vi "PulseProtocol.vi"(11 "Array":string[](array[string])) -> (0 "y2Pulse":i32, 1 "y1Pulse":i32, 2 "xPulse":i32, 3 "modePulse":string)   [LabVIEW 2018]
uses:
  Global Variables.vi
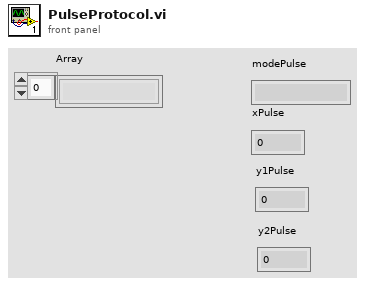
[diagram p1: front panel]
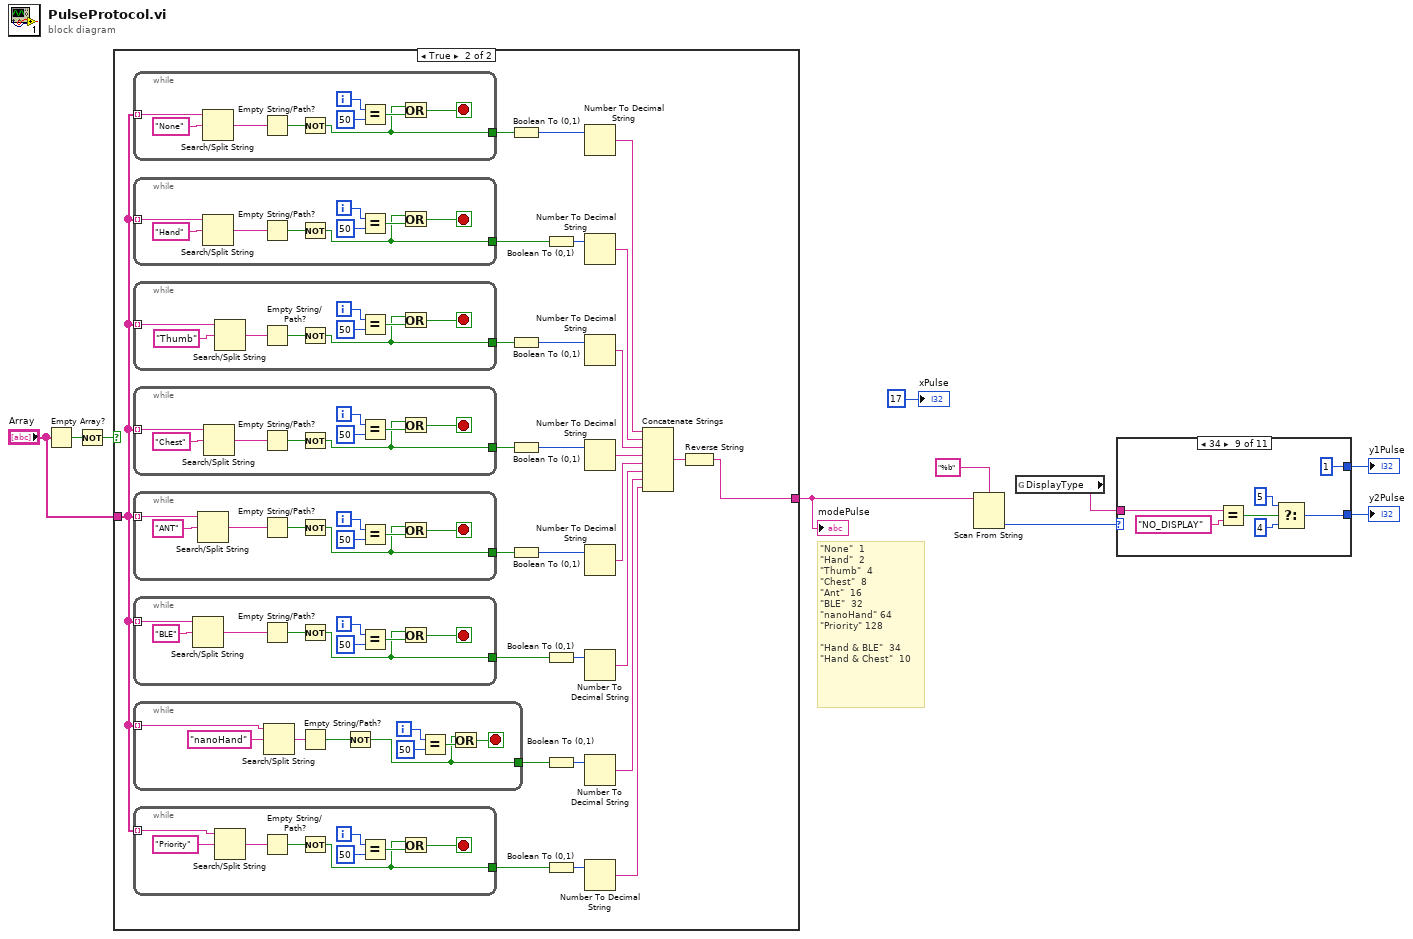
[diagram p0: block diagram]
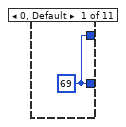
[diagram p2: hidden frame]
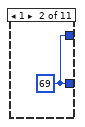
[diagram p3: hidden frame]
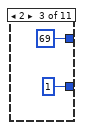
[diagram p4: hidden frame]
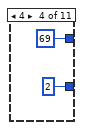
[diagram p5: hidden frame]
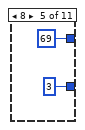
[diagram p6: hidden frame]
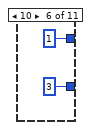
[diagram p7: hidden frame]
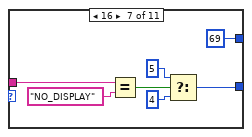
[diagram p8: hidden frame]
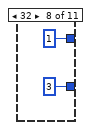
[diagram p9: hidden frame]
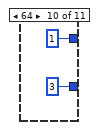
[diagram p10: hidden frame]
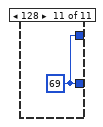
[diagram p11: hidden frame]
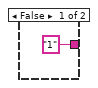
[diagram p12: hidden frame]
diagram:
  # "\"None\"\t\t1\n\"Hand\"\t\t2\n\"Thumb\"\t\t4\n\"Chest\"\t\t8\n\"Ant\"\t\t16\n\"BLE\"\t\t32\n\"nanoHand\"\t64\n\"Priority\"\t128\n\n\"Hand & BLE\"\t\t34\n\"Hand & Chest\"\t\t10"
  n1 = Empty Array?(array="Array") -> (empty?=w8:bool)
  n2 = Not(x=w8) -> (.not. x?=w9:bool)
  n3 = case shown="True" w9 {
    tunnel: "Array" -> [_ w16]
    tunnel: ["1" w12] -> w7
    frame False {
    }
    frame True {
      n4 = while {
        tunnel: w16 -> [w106] mode=indexing
        tunnel: [w102] -> w13
        i -> [w110]
        stop <- w108 stop-if-true
        n5 = Search/Split String(string=w106, search string/char (-)="None") -> (match + rest of string=w103:string)  [unwired: 1 in, 2 out]
        n6 = Empty String/Path?(string/path=w103) -> (empty?=w104:bool)
        n7 = Not(x=w104) -> (.not. x?=w102:bool)
        n8 = Equal?(x=w110, y=50) -> (x = y?=w107:bool)
        n9 = Or(x=w102, y=w107) -> (x .or. y?=w108:bool)
      }
      n10 = while {
        tunnel: w16 -> [w97] mode=indexing
        tunnel: [w93] -> w14
        i -> [w101]
        stop <- w99 stop-if-true
        n11 = Search/Split String(string=w97, search string/char (-)="Hand") -> (match + rest of string=w94:string)  [unwired: 1 in, 2 out]
        n12 = Empty String/Path?(string/path=w94) -> (empty?=w95:bool)
        n13 = Not(x=w95) -> (.not. x?=w93:bool)
        n14 = Equal?(x=w101, y=50) -> (x = y?=w98:bool)
        n15 = Or(x=w93, y=w98) -> (x .or. y?=w99:bool)
      }
      n16 = while {
        tunnel: w16 -> [w88] mode=indexing
        tunnel: [w84] -> w35
        i -> [w92]
        stop <- w90 stop-if-true
        n17 = Search/Split String(string=w88, search string/char (-)="Thumb") -> (match + rest of string=w85:string)  [unwired: 1 in, 2 out]
        n18 = Empty String/Path?(string/path=w85) -> (empty?=w86:bool)
        n19 = Not(x=w86) -> (.not. x?=w84:bool)
        n20 = Equal?(x=w92, y=50) -> (x = y?=w89:bool)
        n21 = Or(x=w84, y=w89) -> (x .or. y?=w90:bool)
      }
      n22 = while {
        tunnel: w16 -> [w79] mode=indexing
        tunnel: [w75] -> w29
        i -> [w83]
        stop <- w81 stop-if-true
        n23 = Search/Split String(string=w79, search string/char (-)="Chest") -> (match + rest of string=w76:string)  [unwired: 1 in, 2 out]
        n24 = Empty String/Path?(string/path=w76) -> (empty?=w77:bool)
        n25 = Not(x=w77) -> (.not. x?=w75:bool)
        n26 = Equal?(x=w83, y=50) -> (x = y?=w80:bool)
        n27 = Or(x=w75, y=w80) -> (x .or. y?=w81:bool)
      }
      n28 = while {
        tunnel: w16 -> [w70] mode=indexing
        tunnel: [w66] -> w28
        i -> [w74]
        stop <- w72 stop-if-true
        n29 = Search/Split String(string=w70, search string/char (-)="ANT") -> (match + rest of string=w67:string)  [unwired: 1 in, 2 out]
        n30 = Empty String/Path?(string/path=w67) -> (empty?=w68:bool)
        n31 = Not(x=w68) -> (.not. x?=w66:bool)
        n32 = Equal?(x=w74, y=50) -> (x = y?=w71:bool)
        n33 = Or(x=w66, y=w71) -> (x .or. y?=w72:bool)
      }
      n34 = while {
        tunnel: w16 -> [w61] mode=indexing
        tunnel: [w57] -> w27
        i -> [w65]
        stop <- w63 stop-if-true
        n35 = Search/Split String(string=w61, search string/char (-)="BLE") -> (match + rest of string=w58:string)  [unwired: 1 in, 2 out]
        n36 = Empty String/Path?(string/path=w58) -> (empty?=w59:bool)
        n37 = Not(x=w59) -> (.not. x?=w57:bool)
        n38 = Equal?(x=w65, y=50) -> (x = y?=w62:bool)
        n39 = Or(x=w57, y=w62) -> (x .or. y?=w63:bool)
      }
      n40 = while {
        tunnel: w16 -> [w52] mode=indexing
        tunnel: [w48] -> w26
        i -> [w56]
        stop <- w54 stop-if-true
        n41 = Search/Split String(string=w52, search string/char (-)="nanoHand") -> (match + rest of string=w49:string)  [unwired: 1 in, 2 out]
        n42 = Empty String/Path?(string/path=w49) -> (empty?=w50:bool)
        n43 = Not(x=w50) -> (.not. x?=w48:bool)
        n44 = Equal?(x=w56, y=50) -> (x = y?=w53:bool)
        n45 = Or(x=w48, y=w53) -> (x .or. y?=w54:bool)
      }
      n46 = while {
        tunnel: w16 -> [w43] mode=indexing
        tunnel: [w39] -> w25
        i -> [w47]
        stop <- w45 stop-if-true
        n47 = Search/Split String(string=w43, search string/char (-)="Priority") -> (match + rest of string=w40:string)  [unwired: 1 in, 2 out]
        n48 = Empty String/Path?(string/path=w40) -> (empty?=w41:bool)
        n49 = Not(x=w41) -> (.not. x?=w39:bool)
        n50 = Equal?(x=w47, y=50) -> (x = y?=w44:bool)
        n51 = Or(x=w39, y=w44) -> (x .or. y?=w45:bool)
      }
      n52 = Boolean To (0,1)(Boolean=w13) -> (0, 1=w36:i16)
      n53 = Boolean To (0,1)(Boolean=w35) -> (0, 1=w38:i16)
      n54 = Boolean To (0,1)(Boolean=w29) -> (0, 1=w34:i16)
      n55 = Boolean To (0,1)(Boolean=w28) -> (0, 1=w33:i16)
      n56 = Boolean To (0,1)(Boolean=w14) -> (0, 1=w37:i16)
      n57 = Boolean To (0,1)(Boolean=w27) -> (0, 1=w32:i16)
      n58 = Boolean To (0,1)(Boolean=w26) -> (0, 1=w31:i16)
      n59 = Boolean To (0,1)(Boolean=w25) -> (0, 1=w30:i16)
      n60 = Number To Decimal String(number=w36) -> (decimal integer string=w17:string)  [unwired: 1 in]
      n61 = Number To Decimal String(number=w37) -> (decimal integer string=w18:string)  [unwired: 1 in]
      n62 = Number To Decimal String(number=w38) -> (decimal integer string=w19:string)  [unwired: 1 in]
      n63 = Number To Decimal String(number=w34) -> (decimal integer string=w20:string)  [unwired: 1 in]
      n64 = Number To Decimal String(number=w33) -> (decimal integer string=w21:string)  [unwired: 1 in]
      n65 = Number To Decimal String(number=w32) -> (decimal integer string=w22:string)  [unwired: 1 in]
      n66 = Number To Decimal String(number=w31) -> (decimal integer string=w23:string)  [unwired: 1 in]
      n67 = Number To Decimal String(number=w30) -> (decimal integer string=w24:string)  [unwired: 1 in]
      n68 = Concatenate Strings(w17, w18, w19, w20, w21, w22, w23, w24) -> (w15:string)
      n69 = Reverse String(1:w15) -> (0:w12:string)
    }
  }
  "modePulse" <- w7
  n70 = Scan From String(format string="%b", input string=w7) -> (output 1=w3:i32)  [unwired: 3 in, 3 out]
  n71 = global read "Global Variables.vi" "DisplayType"() -> (w2:string)
  n72 = case shown="34" w3 {
    tunnel: [w111 w112 1 2 3 3 w122 3 w132 3 w139] -> w4
    tunnel: [w111 w112 69 69 69 1 69 1 1 1 w139] -> w5
    tunnel: w2 -> [_ _ _ _ _ _ w121 _ w133 _ _]
    frame 0, Default {
      w111 = 69
    }
    frame 1 {
      w112 = 69
    }
    frame 2 {
    }
    frame 4 {
    }
    frame 8 {
    }
    frame 10 {
    }
    frame 16 {
      n73 = Equal?(x=w121, y="NO_DISPLAY") -> (x = y?=w126:bool)
      n74 = Select(t=5, s=w126, f=4) -> (s? t:f=w122:i32)
    }
    frame 32 {
    }
    frame 34 {
      n75 = Equal?(x=w133, y="NO_DISPLAY") -> (x = y?=w136:bool)
      n76 = Select(t=5, s=w136, f=4) -> (s? t:f=w132:i32)
    }
    frame 64 {
    }
    frame 128 {
      w139 = 69
    }
  }
  "y1Pulse" <- w5
  "y2Pulse" <- w4
  "xPulse" <- 17
